vi "十进制字符串转十六进制字符串.vi"(1 "字符串":string) -> (0 "电子表格字符串":string)   [LabVIEW 2015]
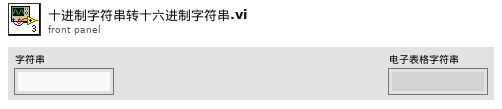
[diagram p1: front panel]
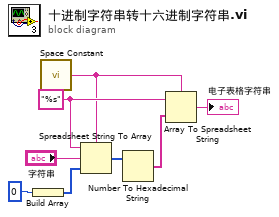
[diagram p0: block diagram]
diagram:
  w3 = "%s"
  n1 = Build Array(0) -> (w6:i32[])
  n2 = call <vilib>:"Space Constant.vi"() -> ("String"=w2:string)
  n3 = Spreadsheet String To Array(delimiter (Tab)=w2, format string=w3, spreadsheet string="字符串", array type (2D Dbl)=w6) -> (array=w5:i32[])
  n4 = Number To Hexadecimal String(2:w5) -> (0:w4:string[])  [unwired: 1 in]
  n5 = Array To Spreadsheet String(delimiter (Tab)=w2, array=w4, 3:w3) -> (spreadsheet string=→"电子表格字符串":string)
